vi "Boolean reference.vi"() -> (0 "Boolean class constant":refnum<vi>)   [LabVIEW 2018, in "Scripting Tools.lvlib"]
uses:
  Scripting Tools.lvlib
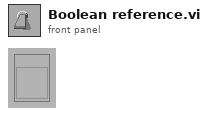
[diagram p1: front panel]
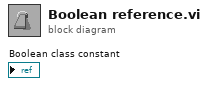
[diagram p0: block diagram]
diagram:
